vi "ArdnoValve2Linx.vi"(6 "Open?":bool, 8 "error in (no error)":errorcluster, 11 "Valve (A1-C8),\n comma separated":string) -> (0 "error out":errorcluster, 2 "Closed State":bool[](array[boolean]), 3 "Linx Port":i32[](array[numeric]))   [LabVIEW 2018, in "Arduino.lvlib"]
uses:
  Arduino.lvlib
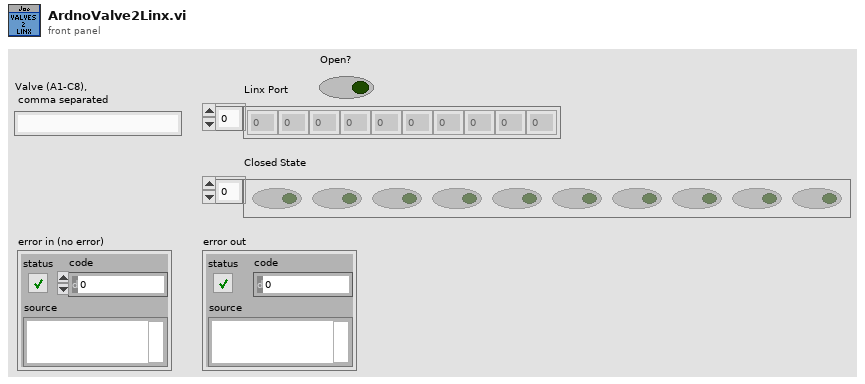
[diagram p1: front panel]
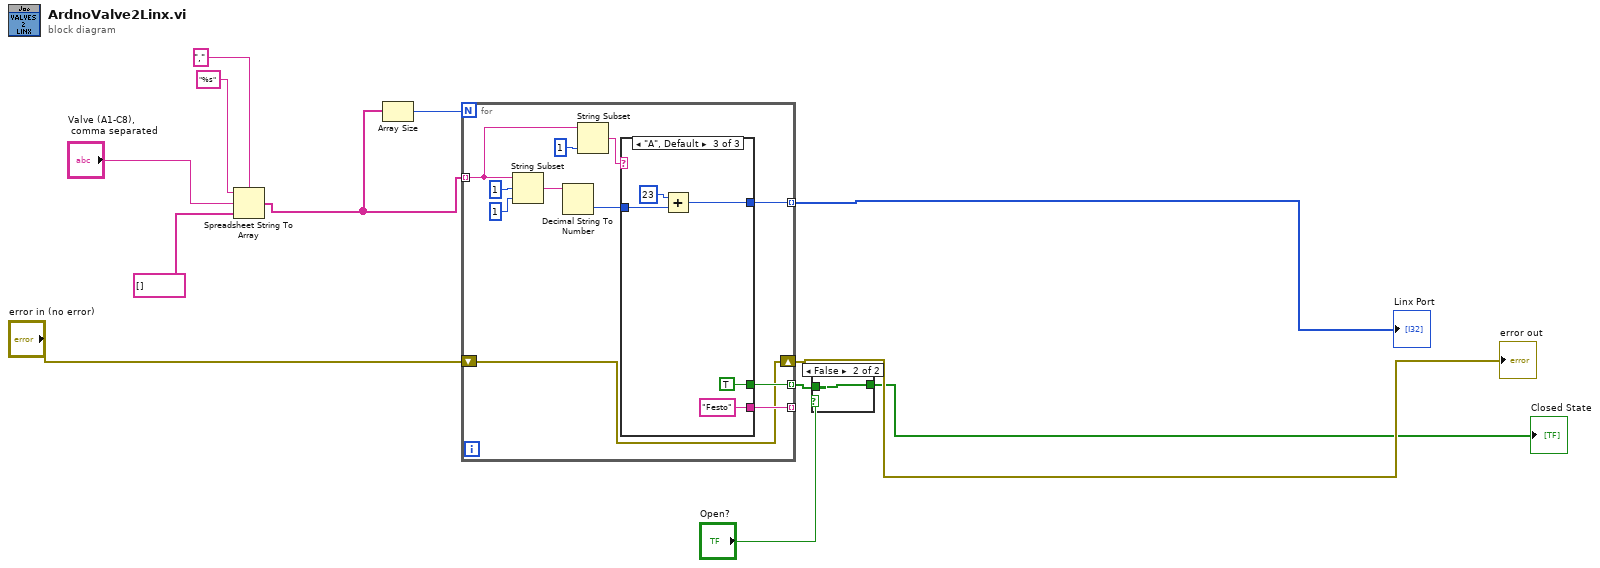
[diagram p0: block diagram]
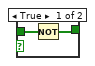
[diagram p2: hidden frame]
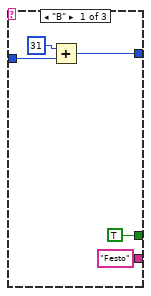
[diagram p3: hidden frame]
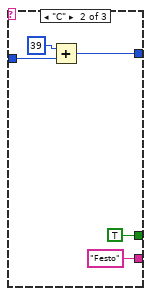
[diagram p4: hidden frame]
diagram:
  n1 = Spreadsheet String To Array(delimiter (Tab)=",", format string="%s", spreadsheet string="Valve (A1-C8),\n comma separated", array type (2D Dbl)=string[] []) -> (array=w7:string[])
  n2 = Array Size(array=w7) -> (size(s)=w11:i32)
  n3 = for {
    N: w11 -> [_]
    tunnel: w7 -> [w20] mode=indexing
    tunnel: [w15] -> w5 mode=indexing
    tunnel: [w16] -> _ mode=indexing
    tunnel: [w14] -> w1 mode=indexing
    shift-right: [w13] -> w3
    shift-left: "error in (no error)" -> [w13]
    n4 = String Subset(string=w20, offset (0)=1, length (rest)=1 ("length (rest)")) -> (substring=w18:string)
    n5 = Decimal String To Number(string=w18) -> (number=w17:i32)  [unwired: 2 in, 1 out]
    n6 = String Subset(string=w20, length (rest)=1 ("length (rest)")) -> (substring=w22:string)  [unwired: 1 in]
    n7 = case shown="\"A\", Default" w22 {
      tunnel: [w27 w32 w37] -> w14
      tunnel: w17 -> [w26 w31 w36]
      tunnel: ["Festo" "Festo" "Festo"] -> w16
      tunnel: [TRUE TRUE TRUE] -> w15
      frame "B" {
        n8 = Add(x=31, y=w26) -> (x+y=w27:i32)
      }
      frame "C" {
        n9 = Add(x=39, y=w31) -> (x+y=w32:i32)
      }
      frame "A", Default {
        n10 = Add(x=23, y=w36) -> (x+y=w37:i32)
      }
    }
  }
  "error out" <- w3
  "Linx Port" <- w1
  n11 = case shown="False" "Open?" {
    tunnel: [w39 w41] -> w2
    tunnel: w5 -> [w40 w41]
    frame True {
      n12 = Not(x=w40) -> (.not. x?=w39:bool[])
    }
    frame False {
    }
  }
  "Closed State" <- w2
